vi "coordinate calculation.vi"() -> ()   [LabVIEW 2026]
uses:
  <vilib>/sklein/WebView2/Webview2 Lib/WebView2 Control Object/WebView2 Control.lvclass
  <vilib>/sklein/WebView2/Libs/Microsoft.Web.WebView2.WinForms.dll
panel:
  in  "stop":bool
  in  "Add Button 3":bool
  in  "Add Button 2":bool
  in  "Add Button 1":bool
  in  "OK Button":bool
  in  "WebView2":refnum<k24>(container)
  out "y":dbl
  out "x":dbl
  in  "x0 base3":dbl=40.1817
  in  "y0 base3":dbl=44.5263
  in  "PLm 3":dbl=32.0
  in  "PL 3":dbl=76.0
  in  "x0 base2":dbl=40.1881
  in  "y0 base2":dbl=44.5192
  in  "PLm 2":dbl=32.0
  in  "PL 2":dbl=74.0
  in  "x0 base1":dbl=40.1915
  in  "y0 base1":dbl=44.5221
  in  "PLm":dbl=32.0
  in  "PL":dbl=72.0
  in  "n":dbl=2.0
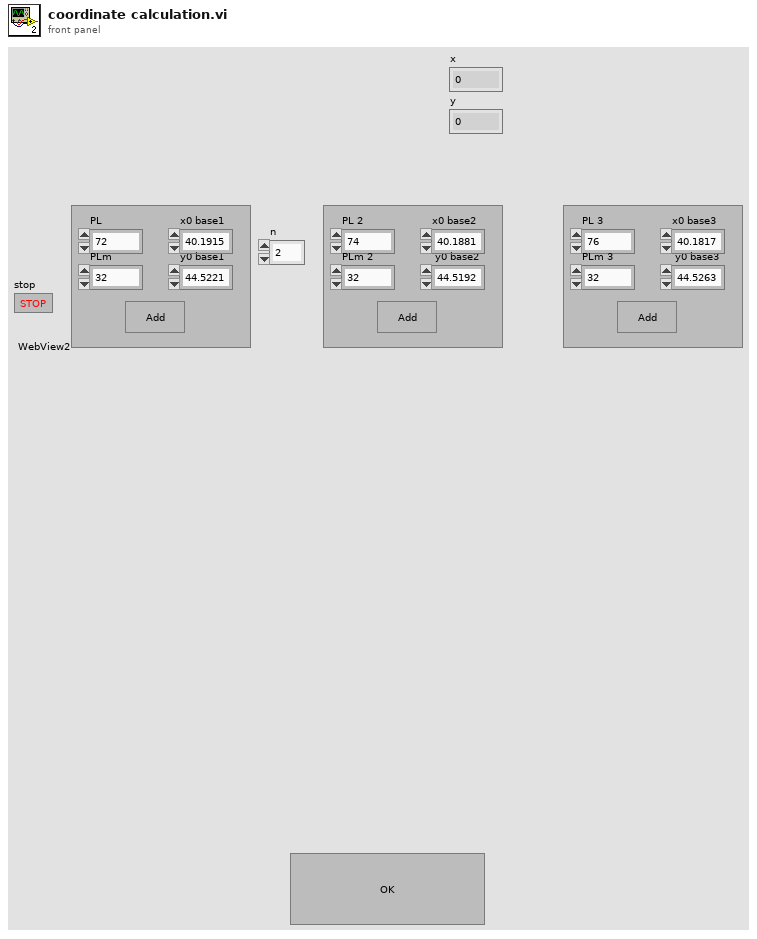
[diagram p1: front panel]
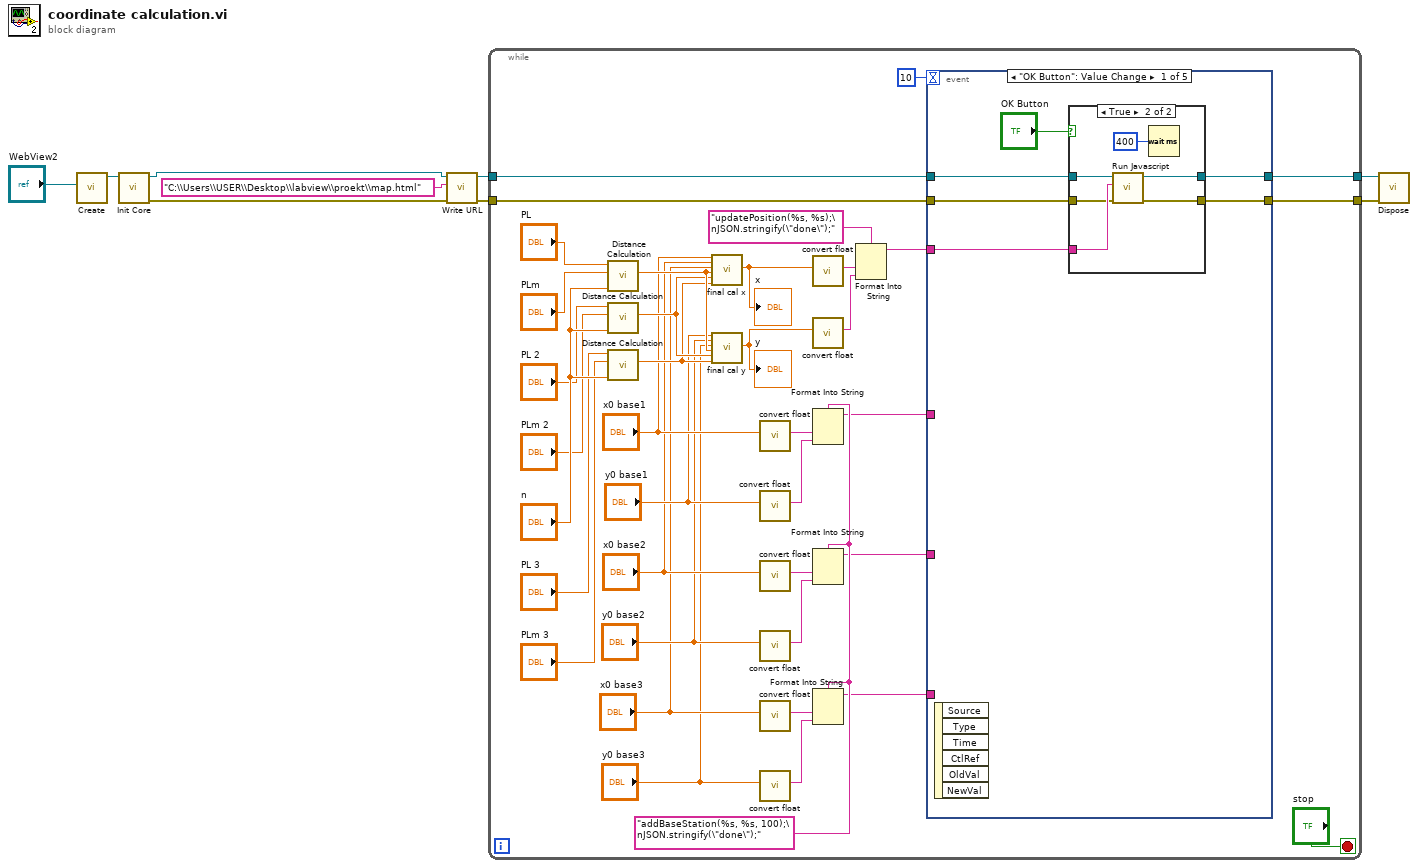
[diagram p0: block diagram]
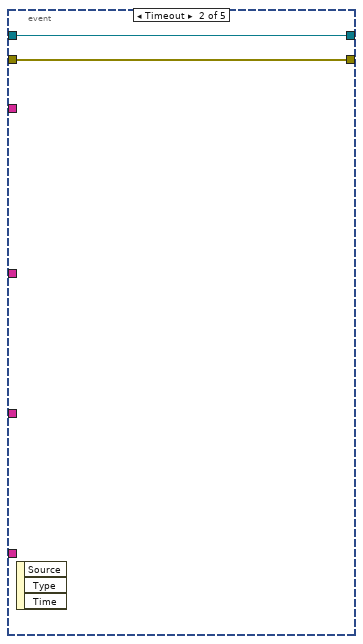
[diagram p3: hidden frame]
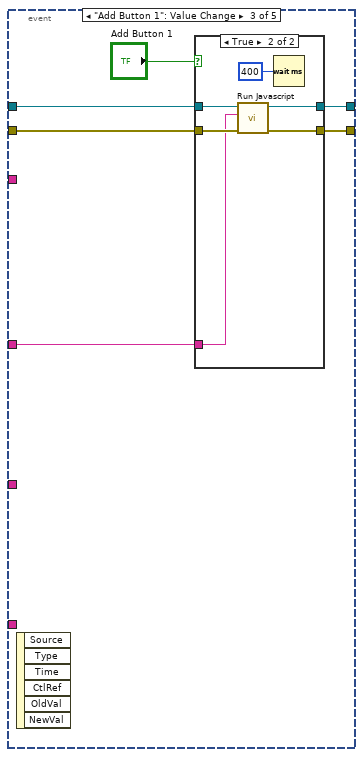
[diagram p4: hidden frame]
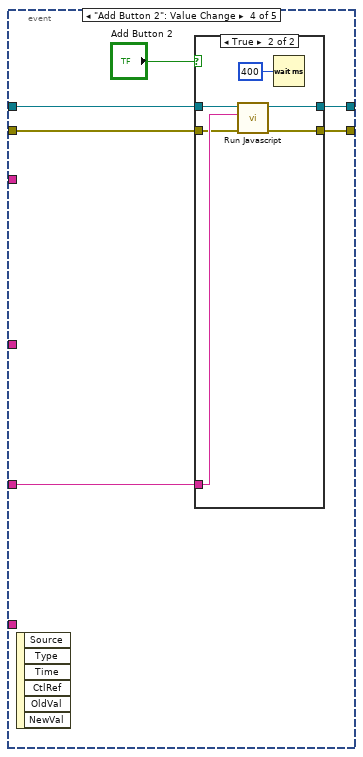
[diagram p6: hidden frame]
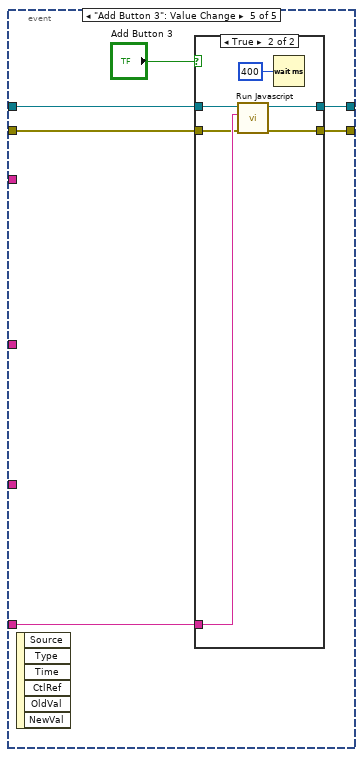
[diagram p8: hidden frame]
diagram:
  n1 = call <vilib>:"Create.vi"("WebView2 Control"="WebView2") -> ("WebView2 Control out"=w7:refnum<class "WebView2 Control.lvclass">)  [unwired: 9 in, 1 out]
  n2 = call <vilib>:"Init Core.vi"("WebView2 Control in"=w7) -> ("error out"=w3:errorcluster, "WebView2 Control out"=w9:refnum<class "WebView2 Control.lvclass">)  [unwired: 9 in]
  n3 = call <vilib>:"Write URL.vi"("error in (no error)"=w3, "uri"="C:\\Users\\USER\\Desktop\\labview\\proekt\\map.html", "WebView2 Control in"=w9) -> ("error out"=w5:errorcluster, "WebView2 Control out"=w4:refnum<class "WebView2 Control.lvclass">)  [unwired: 7 in]
  n4 = while {
    tunnel: w5 -> [w31]
    tunnel: w4 -> [w35]
    tunnel: [w29] -> w2
    tunnel: [w28] -> w1
    stop <- "stop" stop-if-true
    w36 = "addBaseStation(%s, %s, 100);\nJSON.stringify(\"done\");" ("format string")
    n5 = call "Distance Calculation.vi"("n"="n", "PLm"="PLm", "PL"="PL") -> ("d"=w40:dbl)  [unwired: 8 in]
    n6 = call "Distance Calculation.vi"("n"="n", "PLm"="PLm 2", "PL"="PL 2") -> ("d"=w39:dbl)  [unwired: 8 in]
    n7 = call "Distance Calculation.vi"("n"="n", "PLm"="PLm 3", "PL"="PL 3") -> ("d"=w38:dbl)  [unwired: 8 in]
    n8 = call "final cal x.vi"("x0 base 1"="x0 base1", "x0 base 2"="x0 base2", "x0  base 3"="x0 base3", "d1"=w40, "d2"=w39, "d3"=w38) -> ("x"=w11:dbl)  [unwired: 13 in]
    "x" <- w11
    n9 = call "final cal y.vi"("y0 base 1"="y0 base1", "y0 base 2"="y0 base2", "y0  base 3"="y0 base3", "d 1"=w40, "d 2"=w39, "d 3"=w38) -> ("y"=w13:dbl)  [unwired: 13 in]
    "y" <- w13
    n10 = call "convert float.vi"("Numeric"="x0 base1") -> ("result string"=w24:string)  [unwired: 10 in]
    n11 = call "convert float.vi"("Numeric"="y0 base1") -> ("result string"=w23:string)  [unwired: 10 in]
    n12 = call "convert float.vi"("Numeric"="x0 base2") -> ("result string"=w20:string)  [unwired: 10 in]
    n13 = call "convert float.vi"("Numeric"="y0 base2") -> ("result string"=w18:string)  [unwired: 10 in]
    n14 = call "convert float.vi"("Numeric"="x0 base3") -> ("result string"=w16:string)  [unwired: 10 in]
    n15 = call "convert float.vi"("Numeric"="y0 base3") -> ("result string"=w14:string)  [unwired: 10 in]
    n16 = call "convert float.vi"("Numeric"=w11) -> ("result string"=w10:string)  [unwired: 10 in]
    n17 = call "convert float.vi"("Numeric"=w13) -> ("result string"=w12:string)  [unwired: 10 in]
    n18 = Format Into String(format string=w36, w24, w23) -> (resulting string=w33:string)  [unwired: 2 in, 1 out]
    n19 = Format Into String(format string=w36, w20, w18) -> (resulting string=w32:string)  [unwired: 2 in, 1 out]
    n20 = Format Into String(format string=w36, w16, w14) -> (resulting string=w30:string)  [unwired: 2 in, 1 out]
    n21 = Format Into String(format string="updatePosition(%s, %s);\nJSON.stringify(\"done\");", w10, w12) -> (resulting string=w34:string)  [unwired: 2 in, 1 out]
    n22 = event shown="[0] \"OK Button\": Value Change" {
      selector: _ -> [_ _ _ _ _]
      dyn-events: _ -> [_ _ _ _ _]
      timeout: 10 -> [_ _ _ _ _]
      tunnel: w35 -> [w53 w63 w64 w78 w92]
      tunnel: w34 -> [w52 _ _ _ _]
      tunnel: w31 -> [w48 w62 w69 w79 w93]
      tunnel: w33 -> [_ _ w68 _ _]
      tunnel: [w50 w63 w66 w82 w95] -> w29
      tunnel: [w49 w62 w65 w81 w94] -> w28
      tunnel: w32 -> [_ _ _ w83 _]
      tunnel: w30 -> [_ _ _ _ w96]
      event "OK Button": Value Change {
        n23 = event-data() -> ()  [unwired: 1 in, 6 out]
        n24 = case shown="True" "OK Button" {
          tunnel: w53 -> [w55 w61]
          tunnel: [w54 w58] -> w49
          tunnel: [w55 w59] -> w50
          tunnel: w52 -> [_ w60]
          tunnel: w48 -> [w54 w56]
          frame False {
          }
          frame True {
            n25 = call <vilib>:"Run Javascript.vi"("error in (no error)"=w56, "javaScript"=w60, "WebView2 Control in"=w61) -> ("error out"=w58:errorcluster, "WebView2 Control out"=w59:refnum<class "WebView2 Control.lvclass">)  [unwired: 6 in, 1 out]
            n26 = Wait (ms)(milliseconds to wait=u32 400) -> ()  [unwired: 1 out]
          }
        }
      }
      event Timeout {
        n27 = event-data() -> ()  [unwired: 1 in, 3 out]
      }
      event "Add Button 1": Value Change {
        n28 = event-data() -> ()  [unwired: 1 in, 6 out]
        n29 = case shown="True" "Add Button 1" {
          tunnel: w69 -> [w71 w77]
          tunnel: [w71 w74] -> w65
          tunnel: [w70 w75] -> w66
          tunnel: w68 -> [_ w76]
          tunnel: w64 -> [w70 w72]
          frame False {
          }
          frame True {
            n30 = call <vilib>:"Run Javascript.vi"("error in (no error)"=w77, "javaScript"=w76, "WebView2 Control in"=w72) -> ("error out"=w74:errorcluster, "WebView2 Control out"=w75:refnum<class "WebView2 Control.lvclass">)  [unwired: 6 in, 1 out]
            n31 = Wait (ms)(milliseconds to wait=u32 400) -> ()  [unwired: 1 out]
          }
        }
      }
      event "Add Button 2": Value Change {
        n32 = event-data() -> ()  [unwired: 1 in, 6 out]
        n33 = case shown="True" "Add Button 2" {
          tunnel: [w84 w89] -> w81
          tunnel: [w85 w90] -> w82
          tunnel: w83 -> [_ w91]
          tunnel: w79 -> [w84 w87]
          tunnel: w78 -> [w85 w86]
          frame False {
          }
          frame True {
            n34 = call <vilib>:"Run Javascript.vi"("error in (no error)"=w87, "javaScript"=w91, "WebView2 Control in"=w86) -> ("error out"=w89:errorcluster, "WebView2 Control out"=w90:refnum<class "WebView2 Control.lvclass">)  [unwired: 6 in, 1 out]
            n35 = Wait (ms)(milliseconds to wait=u32 400) -> ()  [unwired: 1 out]
          }
        }
      }
      event "Add Button 3": Value Change {
        n36 = event-data() -> ()  [unwired: 1 in, 6 out]
        n37 = case shown="True" "Add Button 3" {
          tunnel: [w98 w103] -> w94
          tunnel: [w99 w104] -> w95
          tunnel: w96 -> [_ w105]
          tunnel: w93 -> [w98 w101]
          tunnel: w92 -> [w99 w100]
          frame False {
          }
          frame True {
            n38 = call <vilib>:"Run Javascript.vi"("error in (no error)"=w101, "javaScript"=w105, "WebView2 Control in"=w100) -> ("error out"=w103:errorcluster, "WebView2 Control out"=w104:refnum<class "WebView2 Control.lvclass">)  [unwired: 6 in, 1 out]
            n39 = Wait (ms)(milliseconds to wait=u32 400) -> ()  [unwired: 1 out]
          }
        }
      }
    }
  }
  n40 = call <vilib>:"Dispose.vi"("error in (no error)"=w1, "WebView2 Control in"=w2) -> ()  [unwired: 9 in, 1 out]
